vi "SegundoEjercicio.vi"() -> ()   [LabVIEW 2022 SP3]
uses:
  <vilib>/Instr/_visa.llb/VISA Configure Serial Port (Instr).vi
panel:
  out "String":string
  out "Thermometer":dbl(slide) scale=0.0..100.0
  out "Gauge":dbl(knob) scale=0.0..100.0
  in  "stop":bool
  in  "VISA resource name":refnum<visa-resource-name>
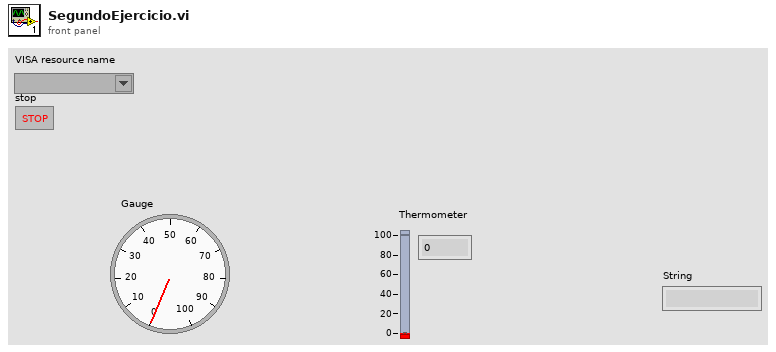
[diagram p1: front panel]
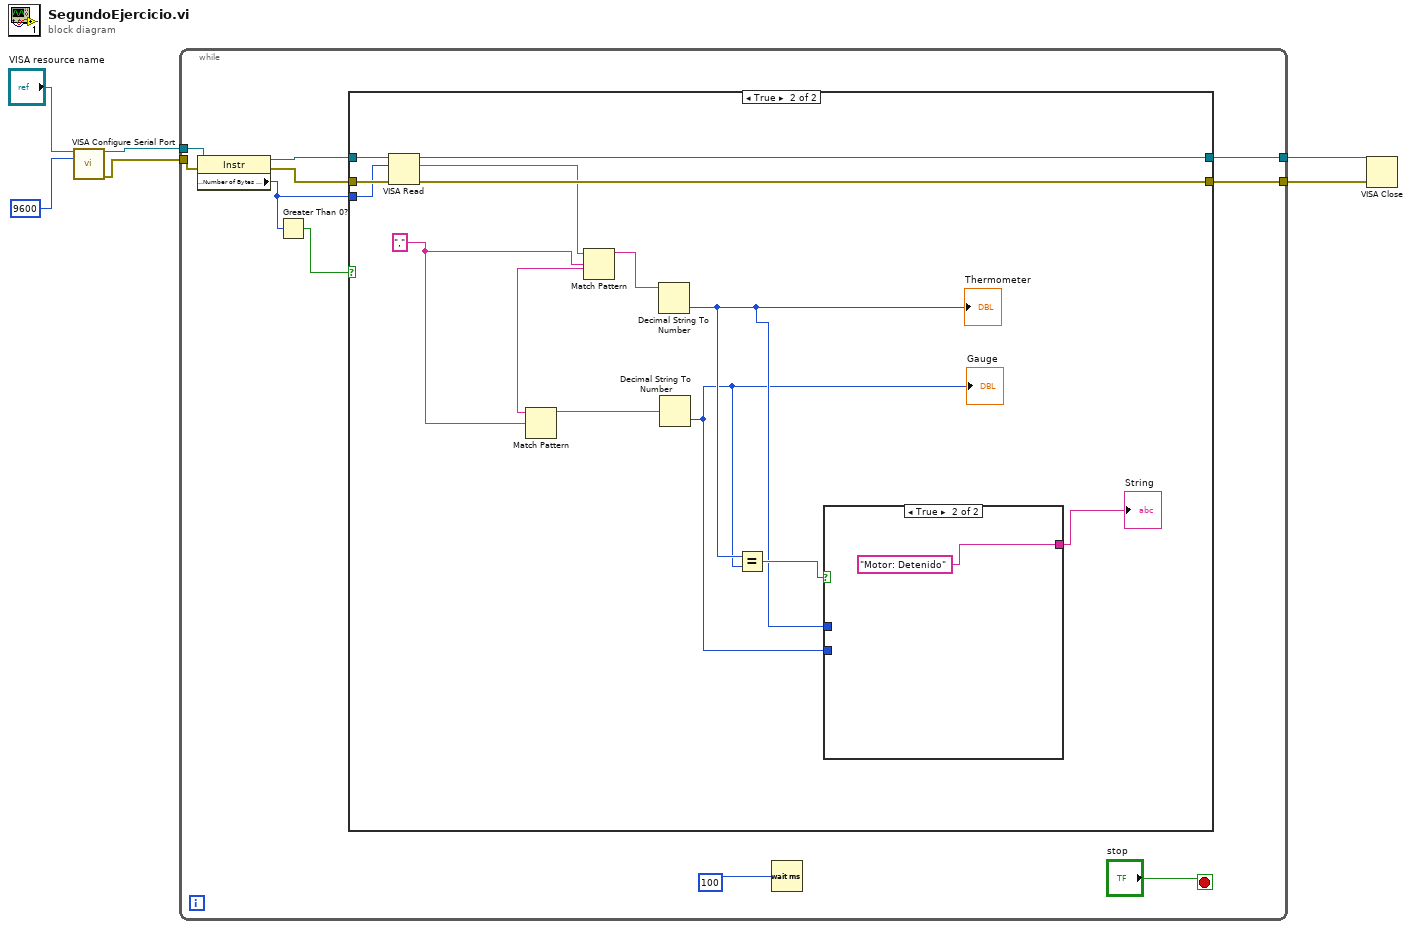
[diagram p0: block diagram]
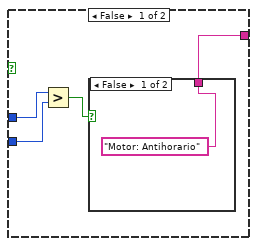
[diagram p3: hidden frame]
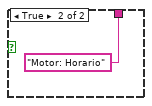
[diagram p4: hidden frame]
diagram:
  n1 = call-poly "VISA Configure Serial Port"("VISA resource name"="VISA resource name", "baud rate (9600)"=u32 9600) -> ("VISA resource name out"=w6:refnum<visa-resource-name>, "error out"=w4:errorcluster)  [unwired: 12 in]
  n2 = while {
    tunnel: w6 -> [w16]
    tunnel: [w14] -> w5
    tunnel: w4 -> [w13]
    tunnel: [w11] -> w3
    stop <- "stop" stop-if-true
    n3 = property class="Instr"(reference=w16, error in=w13) -> (reference out=w15:refnum<visa-resource-name>, error out=w12:errorcluster, "Serial Settings:Number of Bytes at Serial Port"=w7:u32)
    n4 = Greater Than 0?(x=w7) -> (x > 0?=w9:bool)
    n5 = case shown="True" w9 {
      tunnel: w15 -> [w18 w32]
      tunnel: [w18 w31] -> w14
      tunnel: w12 -> [w17 w30]
      tunnel: [w17 w29] -> w11
      tunnel: w7 -> [_ w19]
      frame False {
      }
      frame True {
        w25 = ","
        n6 = VISA Read(VISA resource name=w32, byte count=w19, error in (no error)=w30) -> (VISA resource name out=w31:refnum<visa-resource-name>, read buffer=w28:string, error out=w29:errorcluster)  [unwired: 1 out]
        n7 = Match Pattern(string=w28, regular expression=w25) -> (before substring=w27:string, after substring=w26:string)  [unwired: 1 in, 2 out]
        n8 = Match Pattern(string=w26, regular expression=w25) -> (before substring=w24:string)  [unwired: 1 in, 3 out]
        n9 = Decimal String To Number(string=w27) -> (number=w22:i32)  [unwired: 2 in, 1 out]
        "Thermometer" <- w22
        n10 = Decimal String To Number(string=w24) -> (number=w21:i32)  [unwired: 2 in, 1 out]
        "Gauge" <- w21
        n11 = Equal?(x=w22, y=w21) -> (x = y?=w23:bool)
        n12 = case shown="True" w23 {
          tunnel: [w33 "Motor: Detenido"] -> w20
          tunnel: w22 -> [w36 _]
          tunnel: w21 -> [w35 _]
          frame False {
            n13 = Greater?(x=w36, y=w35) -> (0:w34:bool)
            n14 = case shown="False" w34 {
              tunnel: ["Motor: Antihorario" "Motor: Horario"] -> w33
              frame False {
              }
              frame True {
              }
            }
          }
          frame True {
          }
        }
        "String" <- w20
      }
    }
    n15 = Wait (ms)(milliseconds to wait=u32 100) -> ()  [unwired: 1 out]
  }
  n16 = VISA Close(VISA resource name=w5, error in (no error)=w3) -> ()  [unwired: 1 out]
